vi "Helper - ExitLine to Wpts.vi"(6 "North In":dbl, 7 "Next Point":T1 {"East" format="%#_5g"}, 9 "East In":dbl, 10 "Best Angle":dbl, 11 "Distance":dbl) -> (3 "Point on Line":dbl[][](array[numeric]))   [LabVIEW 2011]
doc: "This VI creates 5 points on two differents lines. Those lines are in a certain angle (45/-45 deg off the line Startpoint-Endpoint), starting at the endpoint. \nThe 5 points on each line divide the line with a length that is equal to the distance SP - EP into five qual parts. \nAfter the points are created, the VI compares both lines and selects the one that is further away from the next waypoint. This ensures, that the point is created on the right side for the desired buoy rounding direction.\nThe output is a 2D array with five rows for each point and two colums for X and Y position of the points."
uses:
  2 Typedefs/Velocity.ctl
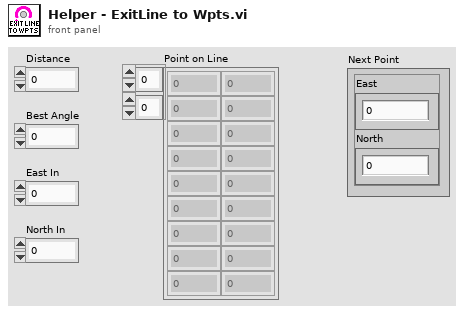
[diagram p1: front panel]
types:
  T1 = typedef "Velocity.ctl" = cluster{"East":dbl, "North":dbl}
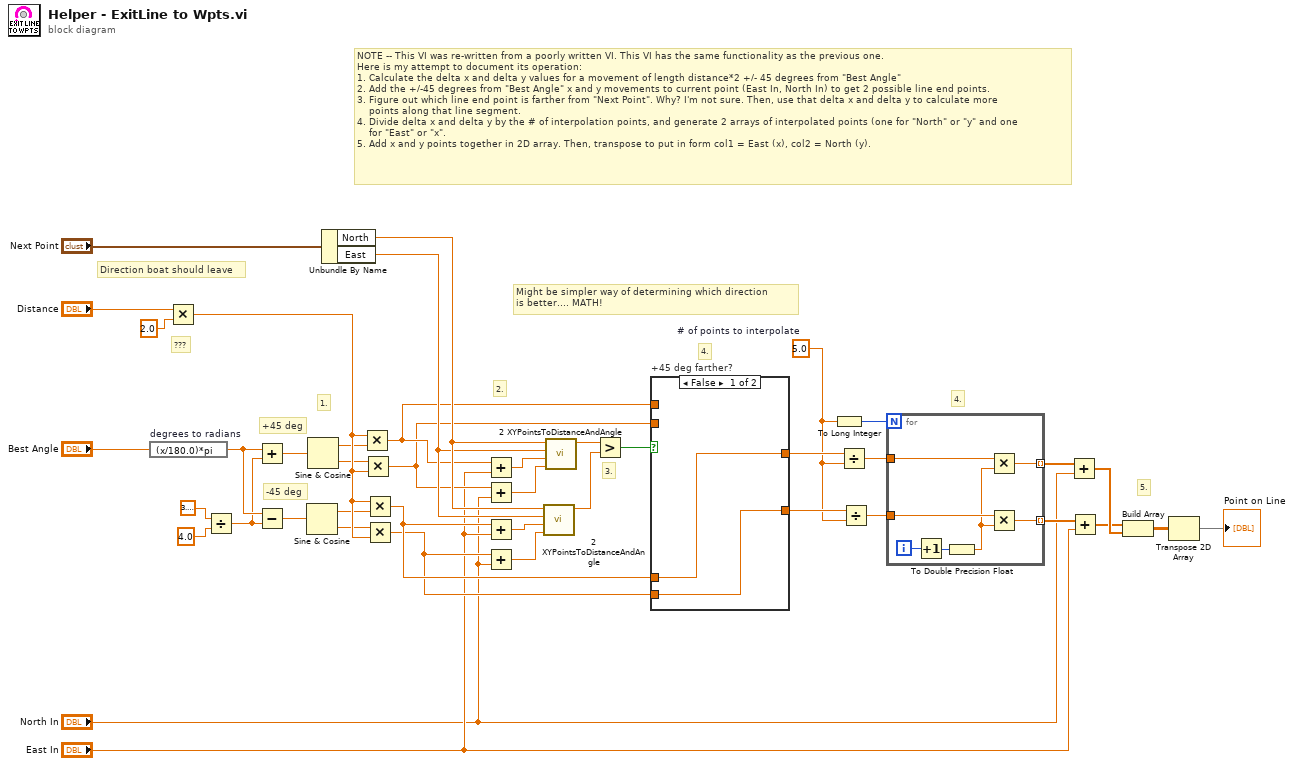
[diagram p0: block diagram]
diagram:
  w20 = 5.0  # # of points to interpolate
  # "5."
  # "4."
  # "4."
  # "3."
  # "2."
  # "1."
  # "NOTE -- This VI was re-written from a poorly written VI. This VI has the same functionality as the previous one.\nHere is my attempt to document its operation: \n1. Calculate the delta x and delta y values for a movement of length distance*2 +/- 45 degrees from \"Best Angle\"\n2. Add the +/-45 degrees from \"Best Angle\" x and y movements to current point (East In, North In) to get 2 possible line end points.\n3. Figure out which line end point is farther from \"Next Point\". Why? I'm not sure. Then, use that delta x and delta y to calculate more\n    points along that line segment.\n4. Divide delta x and delta y by the # of interpolation points, and generate 2 arrays of interpolated points (one for \"North\" or \"y\" and one\n    for \"East\" or \"x\".\n5. Add x and y points together in 2D array. Then, transpose to put in form col1 = East (x), col2 = North (y)."
  # "Might be simpler way of determining which direction\nis better.... MATH!"
  # "-45 deg"
  # "+45 deg"
  # "???"
  # "Direction boat should leave"
  n1 = expression code="(x/180.0)*pi" "degrees to radians"("Best Angle") -> (w39:dbl)
  n2 = Multiply(x="Distance", y=2.0) -> (x*y=w35:dbl)
  n3 = Divide(x=3.141592653589793, y=4.0) -> (x/y=w38:dbl)
  n4 = Add(x=w39, y=w38) -> (x+y=w37:dbl)
  n5 = Subtract(x=w39, y=w38) -> (x-y=w36:dbl)
  n6 = Sine & Cosine(0:w36) -> (1:w27:dbl, 2:w26:dbl)
  n7 = Sine & Cosine(0:w37) -> (1:w29:dbl, 2:w28:dbl)
  n8 = Unbundle By Name("Next Point") -> ("North"=w34:dbl, "East"=w33:dbl)
  n9 = Multiply(x=w35, y=w29) -> (x*y=w15:dbl)
  n10 = Multiply(x=w28, y=w35) -> (x*y=w11:dbl)
  n11 = Multiply(x=w35, y=w27) -> (x*y=w10:dbl)
  n12 = Multiply(x=w26, y=w35) -> (x*y=w9:dbl)
  n13 = Add(x=w15, y="East In") -> (x+y=w16:dbl)
  n14 = Add(x=w11, y="North In") -> (x+y=w14:dbl)
  n15 = Add(x=w10, y="East In") -> (x+y=w13:dbl)
  n16 = Add(x=w9, y="North In") -> (x+y=w12:dbl)
  n17 = call "2 XYPointsToDistanceAndAngle.vi"("East 2"=w12, "North 2"=w13, "East 1"=w33, "North 1"=w34) -> ("Distance"=w31:dbl)  [unwired: 6 in, 1 out]
  n18 = call "2 XYPointsToDistanceAndAngle.vi"("East 2"=w14, "North 2"=w16, "East 1"=w33, "North 1"=w34) -> ("Distance"=w32:dbl)  [unwired: 6 in, 1 out]
  n19 = Greater?(x=w32, y=w31) -> (0:w30:bool)
  n20 = case "+45 deg farther?" shown="False" w30 {
    tunnel: w15 -> [_ w46]
    tunnel: w11 -> [_ w45]
    tunnel: [w44 w46] -> w25
    tunnel: [w43 w45] -> w24
    tunnel: w10 -> [w44 _]
    tunnel: w9 -> [w43 _]
    frame False {
    }
    frame True {
    }
  }
  n21 = To Long Integer(number=w20) -> (32bit integer=w21:i32)
  n22 = Divide(x=w25, y=w20) -> (x/y=w23:dbl)
  n23 = Divide(x=w24, y=w20) -> (x/y=w22:dbl)
  n24 = for {
    N: w21 -> [_]
    tunnel: w23 -> [w52]
    tunnel: w22 -> [w51]
    tunnel: [w48] -> w19 mode=indexing
    tunnel: [w47] -> w18 mode=indexing
    i -> [w53]
    n25 = Increment(x=w53) -> (x+1=w50:i32)
    n26 = To Double Precision Float(number=w50) -> (double precision float=w49:dbl)
    n27 = Multiply(x=w52, y=w49) -> (x*y=w48:dbl)
    n28 = Multiply(x=w51, y=w49) -> (x*y=w47:dbl)
  }
  n29 = Add(x=w19, y="North In") -> (x+y=w8:dbl[])
  n30 = Add(x=w18, y="East In") -> (x+y=w7:dbl[])
  n31 = Build Array(w7, w8) -> (w17:dbl[][])
  n32 = Transpose 2D Array(2D array=w17) -> (transposed array=→"Point on Line":dbl[][])
